vi "Image2Image.vi"() -> (0 "ErrOut":errorcluster)   [LabVIEW 2014]
doc: "Use this template to build a VI to use as a subVI."
uses:
  <vilib>/vision/NI_Vision_Development_Module.lvlib
panel:
  out "Image":T1(plugin-control)
  in  "ErrIn":errorcluster
  # "Input Parameters"
  # "Output Parameters"
  # "VI Description:\nThis VI is .."
  # ":: MVI Framework V1.0 ::\nAuthor:Gaoke Yang\nEmail: gaoke.yang@yahoo.com\nWeb: www.mvicontrol.com\nCopyright (C) 2013, MVI Technologies All Rights Reserved"
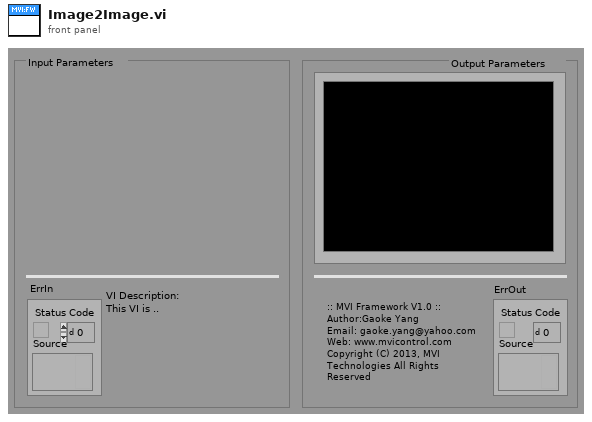
[diagram p1: front panel]
types:
  T1 = typedef "IMAQ Image.ctl" = refnum<image>
  T2 = typedef "Image Type" = u32
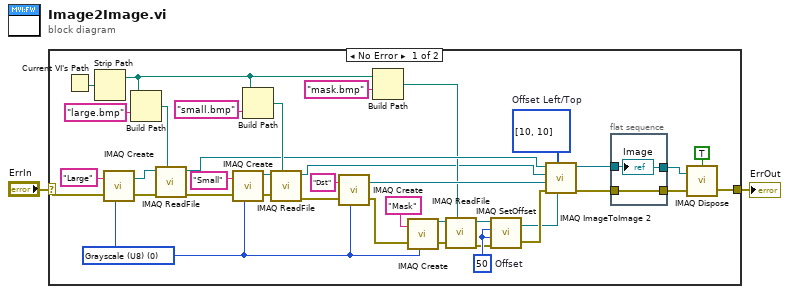
[diagram p0: block diagram]
diagram:
  n1 = case shown="No Error" "ErrIn" {
    selector: "ErrIn" -> [w35 w43]
    tunnel: [w39 w43] -> w2
    frame No Error {
      w15 = 50  # Offset
      w24 = i32[] [10, 10]  # Offset Left/Top
      w3 = T2 0 items=["Grayscale (U8)", "Grayscale (I16)", "Grayscale (SGL)", "Complex (CSG)", "RGB (U32)", "HSL (U32)", "RGB (U64)", "Grayscale (U16)"] ("Image Type")
      n2 = Current VI's Path() -> (path=w37:path)
      n3 = Strip Path(path=w37) -> (stripped path=w18:path)  [unwired: 1 out]
      n4 = call "IMAQ Create"("Image Name"="Large", "Image Type"=w3, "error in (no error)"=w35) -> ("New Image"=w31:T1, "error out"=w11:errorcluster)  [unwired: 2 in]
      n5 = Build Path(base path=w18, name or relative path="large.bmp") -> (appended path=w36:path)
      n6 = call "IMAQ ReadFile"("File Path"=w36, "error in (no error)"=w11, "Image"=w31) -> ("error out"=w9:errorcluster, "Image Out"=w30:T1)  [unwired: 4 in, 3 out]
      n7 = call "IMAQ Create"("Image Name"="Small", "Image Type"=w3, "error in (no error)"=w9) -> ("New Image"=w28:T1, "error out"=w8:errorcluster)  [unwired: 2 in]
      n8 = Build Path(base path=w18, name or relative path="small.bmp") -> (appended path=w32:path)
      n9 = call "IMAQ ReadFile"("File Path"=w32, "error in (no error)"=w8, "Image"=w28) -> ("error out"=w7:errorcluster, "Image Out"=w10:T1)  [unwired: 4 in, 3 out]
      n10 = call "IMAQ Create"("Image Name"="Dst", "Image Type"=w3, "error in (no error)"=w7) -> ("New Image"=w27:T1, "error out"=w6:errorcluster)  [unwired: 2 in]
      n11 = Build Path(base path=w18, name or relative path="mask.bmp") -> (appended path=w17:path)
      n12 = call "IMAQ Create"("Image Name"="Mask", "Image Type"=w3, "error in (no error)"=w6) -> ("New Image"=w16:T1, "error out"=w5:errorcluster)  [unwired: 2 in]
      n13 = call "IMAQ ReadFile"("File Path"=w17, "error in (no error)"=w5, "Image"=w16) -> ("error out"=w13:errorcluster, "Image Out"=w14:T1)  [unwired: 4 in, 3 out]
      n14 = call "IMAQ SetOffset"("error in (no error)"=w13, "Y Offset"=w15, "X Offset"=w15, "Image"=w14) -> ("error out"=w12:errorcluster, "Image Out"=w4:T1)
      n15 = call "IMAQ ImageToImage 2"("Image Mask"=w4, "Offset Left/Top"=w24, "error in (no error)"=w12, "Image Dst"=w27, "Image Src (Small)"=w10, "Image Src (Large)"=w30) -> ("error out"=w21:errorcluster, "Image Dst Out"=w22:T1)  [unwired: 4 in]
      n16 = flat-sequence {
        tunnel: w21 -> [w42]
        tunnel: [w42] -> w26
        tunnel: w22 -> [w41]
        tunnel: [w41] -> w25
        frame #0 {
          "Image" <- w41
        }
      }
      n17 = call "IMAQ Dispose"("All Images? (No)"=TRUE, "Image"=w25, "error in (no error)"=w26) -> ("error out"=w39:errorcluster)  [unwired: 3 in]
    }
    frame Error {
    }
  }
  "ErrOut" <- w2
